vi "Convert Signal Cluster to String Array.vi"(11 "Signal Parameters":T1 {"Byte Order" items=["Little Endian", "Big Endian"]; "Data Type" items=["Signed", "Unsigned", "IEEE Float"]}) -> (3 "Array":string[](array[string]))   [LabVIEW 2015, in "Diagnostics Addon System Explorer.lvlib"]
uses:
  Diagnostics Addon System Explorer.lvlib
  Shared/Signal Parameters.ctl
  Shared/Diagnostics Addon Shared.lvlib
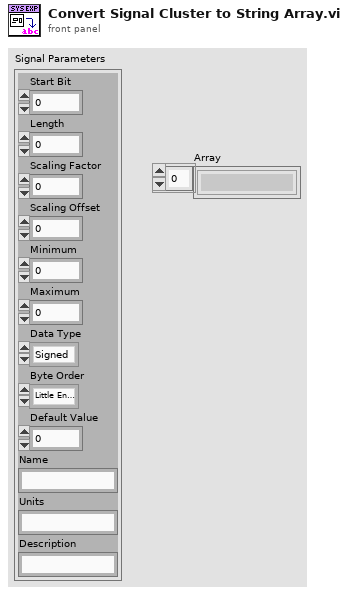
[diagram p1: front panel]
types:
  T1 = typedef "Diagnostics Addon Shared.lvlib/Signal Parameters.ctl" = cluster{"Start Bit":u8, "Length":u8, "Scaling Factor":dbl, "Scaling Offset":dbl, "Minimum":dbl, "Maximum":dbl, "Data Type":u32, "Byte Order":u32, "Default Value":dbl, "Name":string, "Units":string, "Description":string}
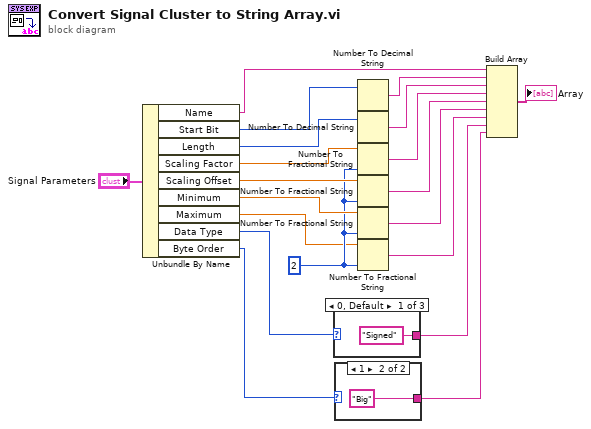
[diagram p0: block diagram]
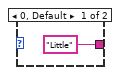
[diagram p2: hidden frame]
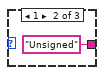
[diagram p3: hidden frame]
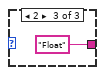
[diagram p4: hidden frame]
diagram:
  w6 = i16 2 ("precision (6)")
  n1 = Unbundle By Name("Signal Parameters") -> ("Name"=w12:string, "Start Bit"=w11:u8, "Length"=w10:u8, "Scaling Factor"=w9:dbl, "Scaling Offset"=w8:dbl, "Minimum"=w7:dbl, "Maximum"=w5:dbl, "Data Type"=w4:u32, "Byte Order"=w2:u32)
  n2 = case shown="0, Default" w4 {
    tunnel: ["Signed" "Unsigned" "Float"] -> w3
    frame 0, Default {
    }
    frame 1 {
    }
    frame 2 {
    }
  }
  n3 = case shown="1" w2 {
    tunnel: ["Little" "Big"] -> w1
    frame 0, Default {
    }
    frame 1 {
    }
  }
  n4 = Number To Decimal String(number=w11) -> (decimal integer string=w13:string)  [unwired: 1 in]
  n5 = Number To Decimal String(number=w10) -> (decimal integer string=w14:string)  [unwired: 1 in]
  n6 = Number To Fractional String(number=w9, precision (6)=w6) -> (F-format string=w15:string)  [unwired: 2 in]
  n7 = Number To Fractional String(number=w8, precision (6)=w6) -> (F-format string=w16:string)  [unwired: 2 in]
  n8 = Number To Fractional String(number=w7, precision (6)=w6) -> (F-format string=w17:string)  [unwired: 2 in]
  n9 = Number To Fractional String(number=w5, precision (6)=w6) -> (F-format string=w18:string)  [unwired: 2 in]
  n10 = Build Array(w12, w13, w14, w15, w16, w17, w18, w3, w1) -> (→"Array":string[])
